vi "Get Read From VS Channel Refs.vi"(8 "error in (no error)":errorcluster, 10 "Refs":T3[](array[typedef]) format="%.0x", 11 "Item Ref in":T3 format="%.0x") -> (0 "error out":errorcluster, 2 "Pairs":cluster{"Refs":T1[], "Values":dbl[]} {"Refs"."Data Reference" format="%.0x"}, 3 "Device Ref out":T3 format="%.0x")   [LabVIEW 2020, in "Instrument Addon System Explorer.lvlib"]
uses:
  Instrument Addon System Explorer.lvlib
  <vilib>/NI VeriStand/Custom Device API/Custom Device Item Ref.ctl
  <vilib>/NI VeriStand/Custom Device API/Block Data Reference.ctl
  <vilib>/NI VeriStand/Custom Device API/Data Reference.ctl
  <vilib>/NI VeriStand/Custom Device API/Data Access Type.ctl
  <vilib>/NI VeriStand/Custom Device API/Custom Device API.lvlib
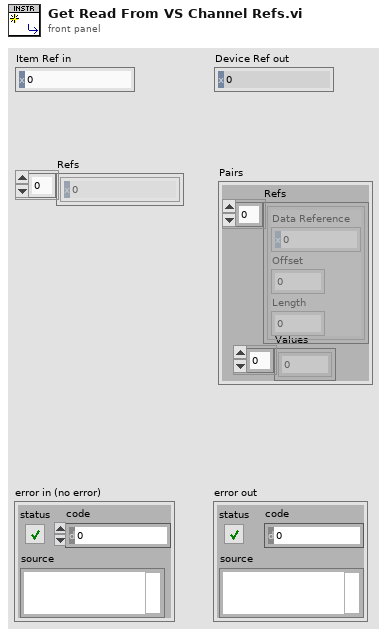
[diagram p1: front panel]
types:
  T1 = typedef "Custom Device API.lvlib/Block Data Reference.ctl" = cluster{"Data Reference":T2, "Offset":u64, "Length":u64}
  T2 = typedef "Custom Device API.lvlib/Data Reference.ctl" = i32
  T3 = typedef "Custom Device API.lvlib/Custom Device Item Ref.ctl" = u64
  T4 = typedef "Custom Device API.lvlib/Data Access Type.ctl" = enum16{"Read", "Write"}
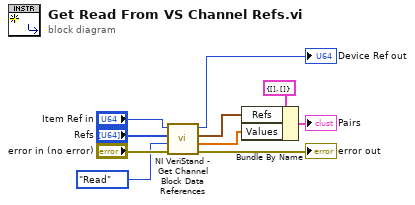
[diagram p0: block diagram]
diagram:
  n1 = call <vilib>:"NI VeriStand - Get Channel Block Data References.vi"("error in (no error)"="error in (no error)", "Access"=Data_Access_Type."Read", "Channel Refs"="Refs", "Device Ref in"="Item Ref in") -> ("error out"=→"error out":errorcluster, "Values Array"=w8:dbl[], "Block Data Refs"=w7:T1[], "Device Ref out"=→"Device Ref out":T3)  [unwired: 4 in]
  n2 = Bundle By Name(cluster=cluster{"Refs":T1[], "Values":dbl[]} {"Refs"=[], "Values"=[]} ("Pairs"), "Refs"=w7, "Values"=w8) -> (→"Pairs":cluster{"Refs":T1[], "Values":dbl[]})
